vi "Slave FPGA Interface.vi"() -> ()   [LabVIEW 2011]
doc: "This VI shows an example of how to implement a closed loop position move using the NI 9505. The position loop is implemented using PID. The output of the loop is used as the command for the current loop, which then sets the PWM duty cycle for the motor. This example assumes that an encoder is connected for position and velocity feedback. This example does not implement advanced motion features such as trajectory generation and splining."
uses:
  <vilib>/LabVIEW Targets/FPGA/cRIO/cRIO-9505/controls.llb/_nicrio_cRIO-9505_DriveStatus.ctl
  <vilib>/Platform/TimedLoop/XDataNode/timing_clust.ctl
  <vilib>/Platform/TimedLoop/XDataNode/nitl_modes.ctl
  <vilib>/Platform/TimedLoop/XDataNode/wakeup.ctl
  <vilib>/LabVIEW Targets/FPGA/cRIO/shared/nicrio_ModuleControls/nicrio_cRIO-9205_VoltageRange.ctl
  <vilib>/LabVIEW Targets/FPGA/cRIO/shared/nicrio_ModuleControls/nicrio_cRIO-9205_TerminalMode.ctl
  <vilib>/LabVIEW Targets/FPGA/cRIO/cRIO-9505/controls.llb/_nicrio_cRIO-9505_DriveDirection.ctl
  Instance           1 55Saved   Position Control (closed loop) - NI 9505 (FPGA) .vi
  <vilib>/rvi/eio/common/nirviEmuTemplateMethod_errors.vi
  Instance           2 55Saved   Position Control (closed loop) - NI 9505 (FPGA) .vi
  <vilib>/rvi/eio/common/nirviEmuTemplatePropertyGet_noerrors.vi
  Instance           3 55Saved   Position Control (closed loop) - NI 9505 (FPGA) .vi
  <vilib>/Platform/TimedLoop/XDataNode/XDataNode.xnode
  <vilib>/eio/EIONode/EIONode.xnode
  <vilib>/eio/EIOMethodNode/EIOMethodNode.xnode
  <vilib>/eio/EIOPropertyNode/EIOPropertyNode.xnode
  <vilib>/Platform/TimedLoop/XDataNode/XDNodeRunTimeDep.lvlib
  <vilib>/rvi/eio/common/nirviEmuTemplatePropertyGet_errors.vi
  <vilib>/rvi/eio/common/nirviEmuTemplatePropertySet_errors.vi
  <vilib>/rvi/eio/common/nirviEmuTemplatePropertySet_noerrors.vi
panel:
  out "Position Error Status":bool
  out "Position Error Read":i16
  out "Current Command":i16
  in  "Position PID Gains":T1={"Kp"=50, "Kd"=1000, "Ki"=0, "ILim"=1000, "Kv"=0, "Vff"=0, "Aff"=0, "Td"=0}
  in  "Position Loop Rate (usec)":u32
  in  "Position Error Limit":i16
  in  "Position Setpoint":i32
  out "ForceSensor AI0-5":fxp<+/-,26,5>[](array[numeric])
  out "FPGA\nError Out":errorcluster
  in  "Force Loop Rate (usec)":u32=50
  out "Vsup Present":bool
  out "Drive Fault":bool
  out "Drive Status":T2=enum."Disabled"
  out "Temp Fault":bool
  in  "Enable\nDrive":bool
  in  "Disable\nDrive":bool
  in  "Reset Position":bool
  in  "Reset Position Value":i32
  out "Encoder Position":i32
  out "ticks/count":u32
  out "Index (Z) Position":i32
  out "counts (no reset)":i32
  in  "Current PI Gains":T3={"Proportional Gain"=20, "Integral Gain"=10, "Derivative Gain"=0}
  in  "Current Limit":i16 caption="Setpoint"
  in  "Current Loop\nRate (usec)":u32=50
  in  "Trig AI":bool
  in  "Current Feedback":i16
  out "Current Loop Output":i16
  # "VI Execution\nThis VI should be run with \"Position Control (closed loop) - NI 9505 (RT).vi\"."
  # "These parameters control the response of the position loop. Position Setpoint is the desired position to go to. Position Error Limit is the maximum allowed error the setpoint and actual position returned by the encoder loop."
  # "These parameters control the response\nof the current loop. The current limit is the \nmaximum current allowed."
  # "Current Loop Parameters"
  # "Use the Reset Position control to reset the quadrature count to the value in Reset Position Value."
  # "These status controls/indicators are used to enable/disable the drive and read fault information."
  # "Drive Status"
  # "Encoder Parameters"
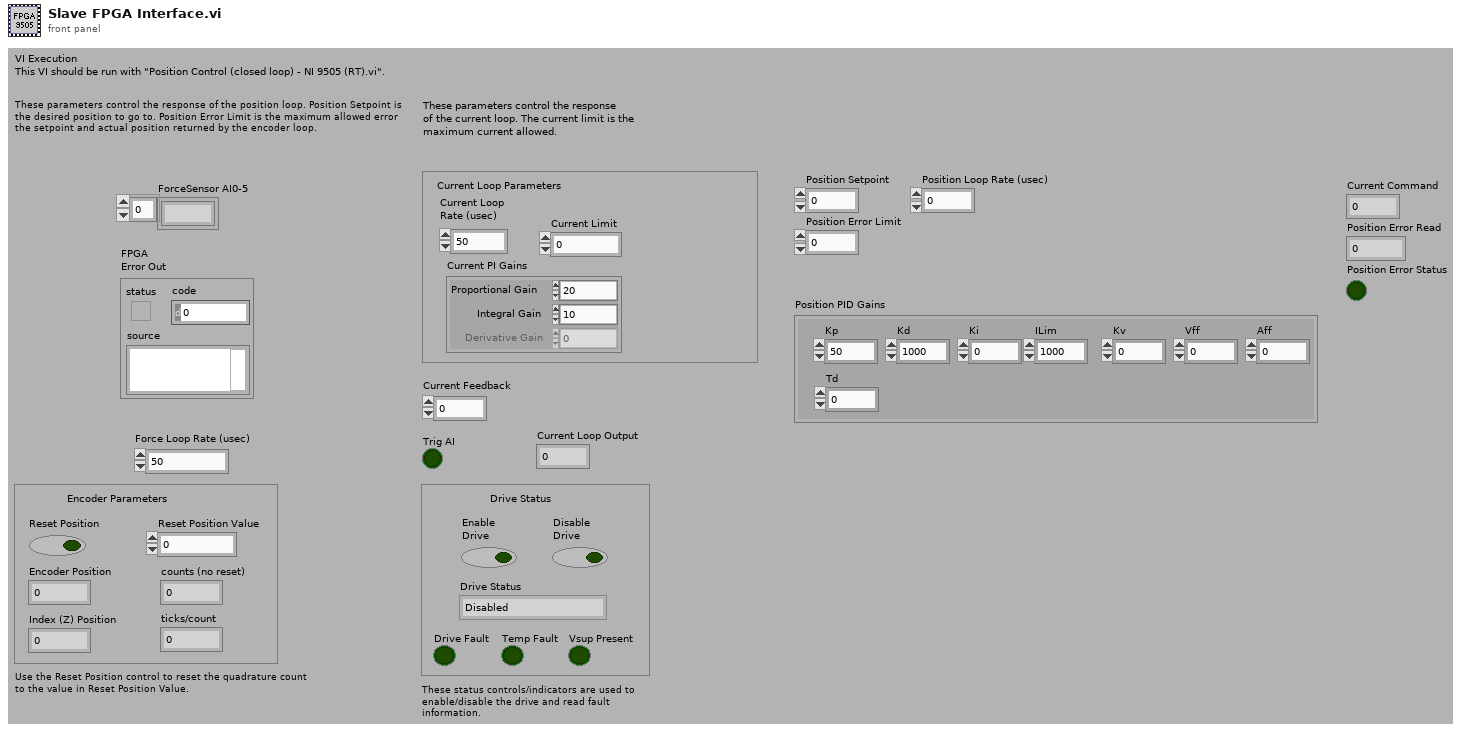
[diagram p1: front panel]
types:
  T1 = cluster{"Kp":i16, "Kd":i16, "Ki":i16, "ILim":i16, "Kv":i16, "Vff":i16, "Aff":i16, "Td":i16}
  T2 = typedef "_nicrio_cRIO-9505_DriveStatus.ctl" = enum8{"Enabled", "Disabled", "Disabled by Drive Fault", "Disabled by Temp. Fault", "Disabled by E-Stop", "Unknown"}
  T3 = cluster{"Proportional Gain":i16, "Integral Gain":i16, "Derivative Gain":i16}
  T4 = typedef "XDNodeRunTimeDep.lvlib/timing_clust.ctl" = cluster{"Expected End [f-1]":u64, "Actual End [f-1]":u64, "Finished Late? [f-1]":bool, "Expected End [i-1]":u64, "Actual End [i-1]":u64, "Finished Late? [i-1]":bool, "Expected Start [i]":u64, "Actual Start [i]":u64, "Expected Start [f]":u64, "Actual Start [f]":u64, "Source Name":string, "Structure Name":string, "Period":i64, "Deadline":i64, "Offset":i64, "Start":i64, "Priority":i32, "Timeout":i32, "Mode":T5, "Wakeup Reason":T6, "Error":errorcluster, "Source Type":string, "Secondary Source Type":string, "Global End Time":u64, "Global Start Time":u64, "Frame Duration":u64, "Iteration Duration":u64, "Assigned CPU":i32, "I/O Scan Engine Mode":u32}
  T5 = typedef "XDNodeRunTimeDep.lvlib/nitl_modes.ctl" = enum32{"No Change", "Process missed periods, maintain original phase", "Discard missed periods, maintain original phase", "Process missed periods, ignore original phase", "Discard missed periods, ignore original phase"}
  T6 = typedef "XDNodeRunTimeDep.lvlib/wakeup.ctl" = enum32{"Normal", "Aborted", "Asynchronous wakeup", "Timing source error", "Timed loop error", "Timeout"}
  T7 = typedef "_nicrio_cRIO-9505_DriveDirection.ctl" = enum8{"Clockwise", "Counterclockwise"}
  T8 = typedef "nicrio_cRIO-9205_VoltageRange.ctl" = enum8{"+/- 10V", "+/- 5V", "+/- 1V", "+/- 200mV"}
  T9 = typedef "nicrio_cRIO-9205_TerminalMode.ctl" = enum8{"RSE", "NRSE", "DIFF"}
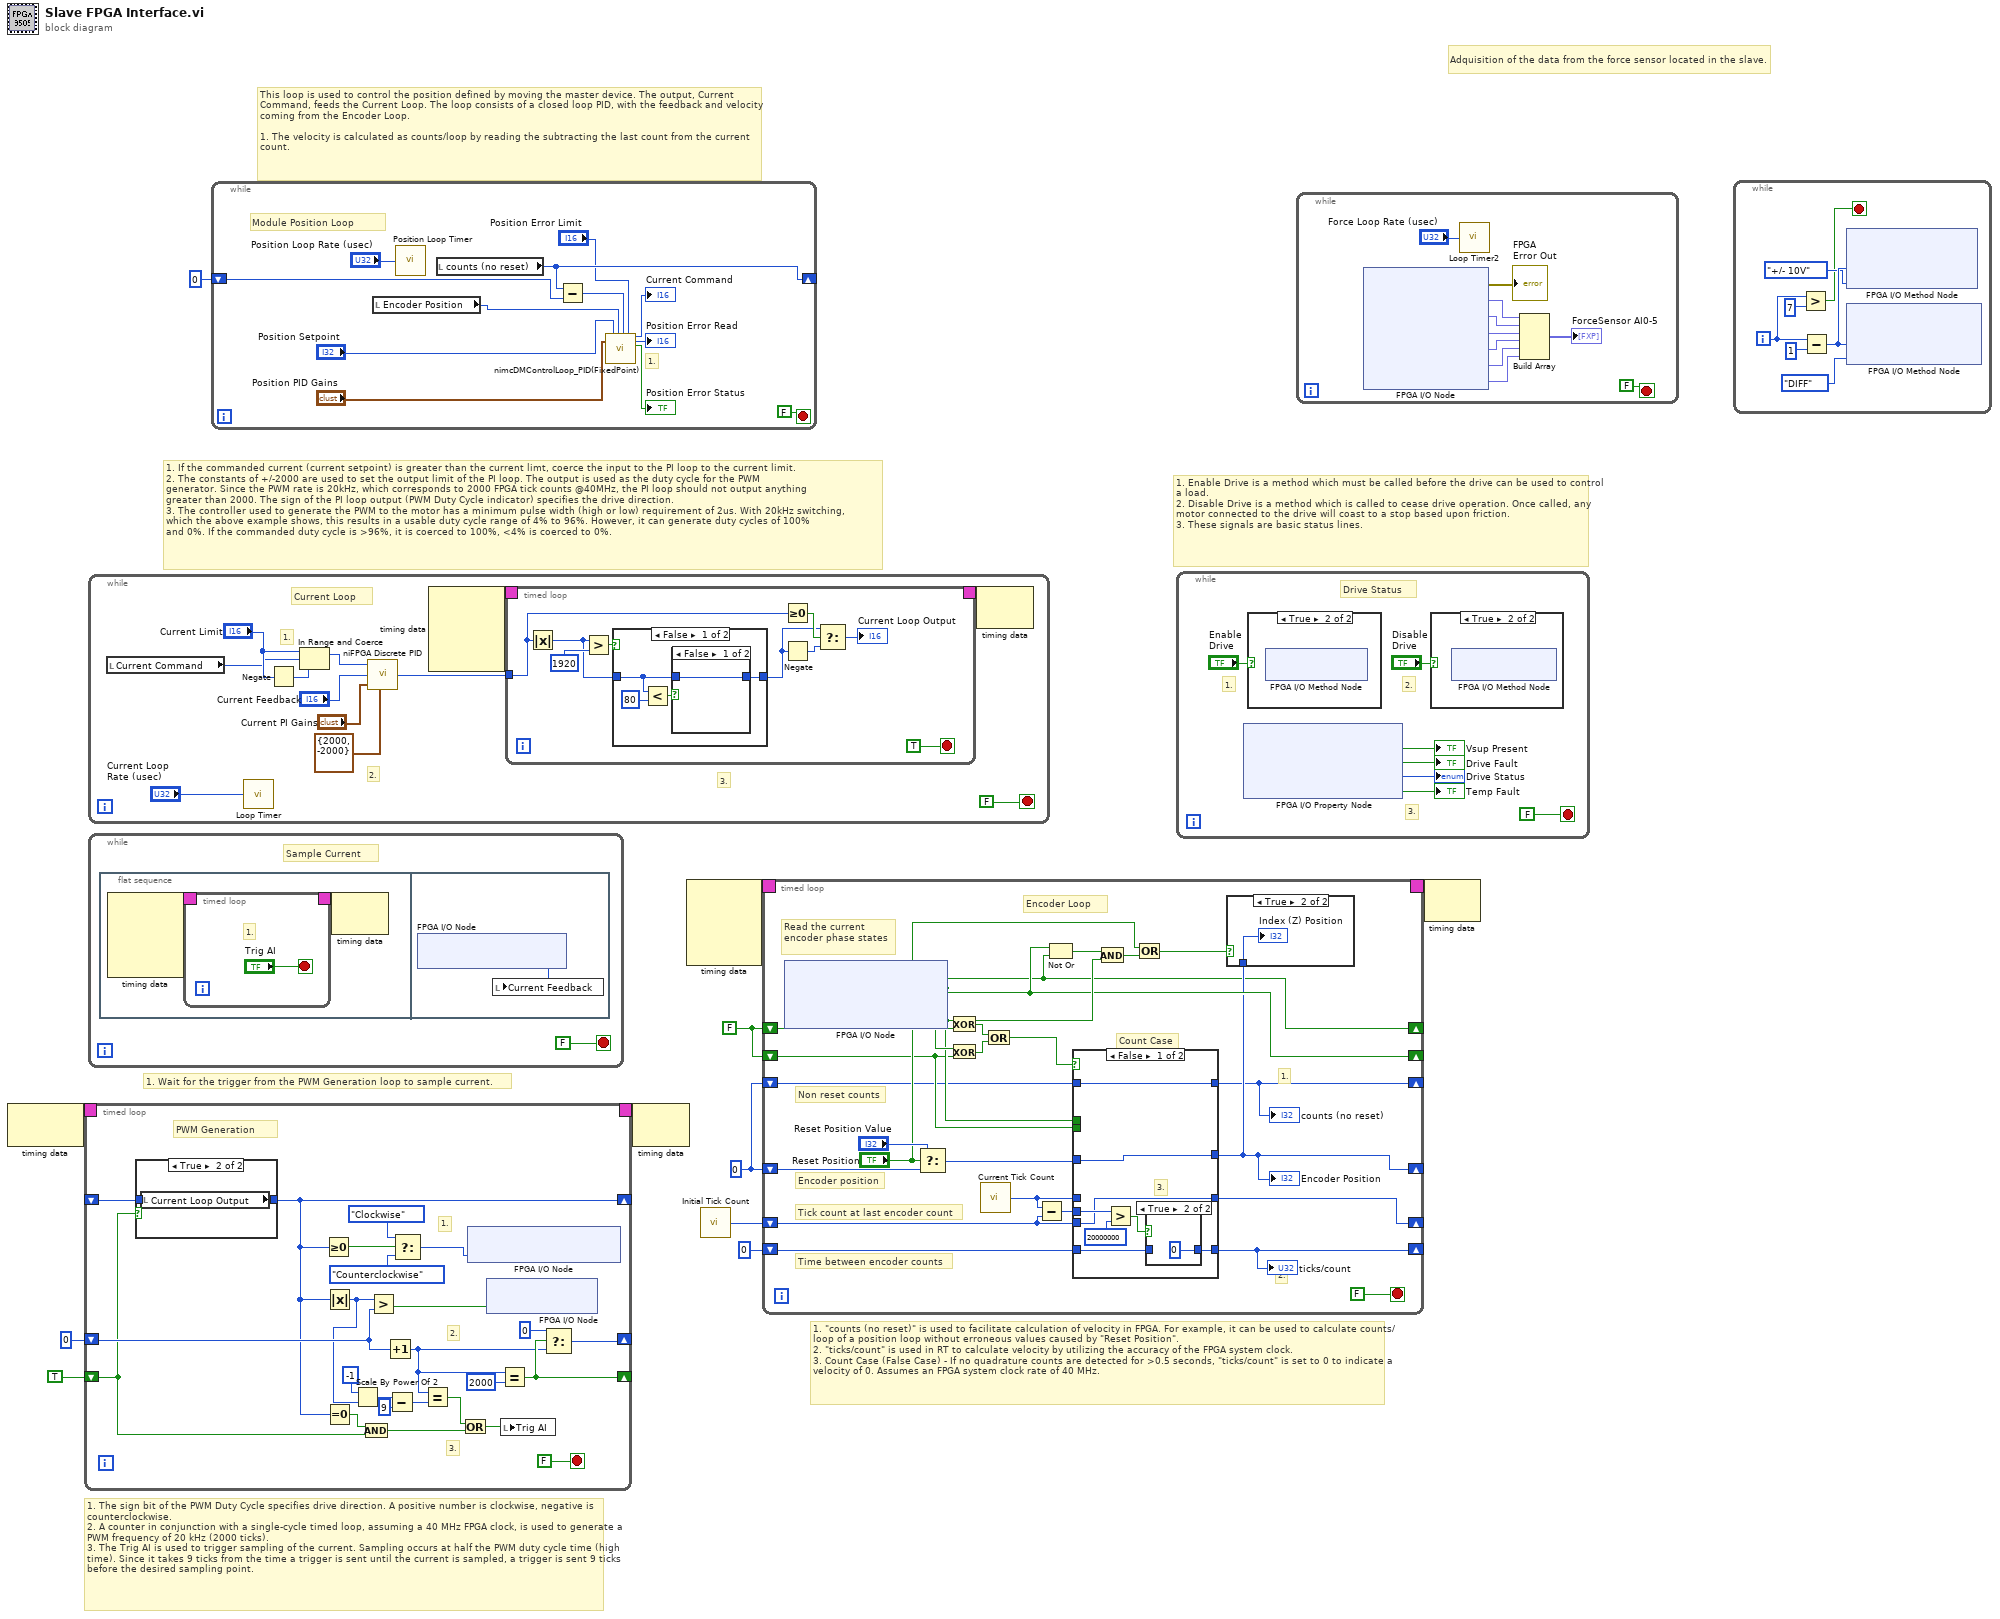
[diagram p0: block diagram]
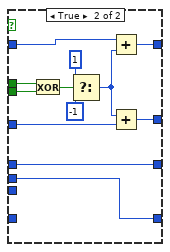
[diagram p4: hidden frame]
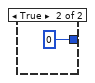
[diagram p6: hidden frame]
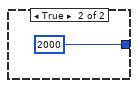
[diagram p7: hidden frame]
diagram:
  w2 = 0 ("Reset Position Value")
  w5 = FALSE ("Encoder Phase A")
  # "This loop is used to control the position defined by moving the master device. The output, Current Command, feeds the Current Loop. The loop consists of a closed loop PID, with the feedback and velocity coming from the Encoder Loop.\n\n1. The velocity is calculated as counts/loop by reading the subtracting the last count from the current count."
  # "Adquisition of the data from the force sensor located in the slave."
  # "1. \"counts (no reset)\" is used to facilitate calculation of velocity in FPGA. For example, it can be used to calculate counts/loop of a position loop without erroneous values caused by \"Reset Position\". \n2. \"ticks/count\" is used in RT to calculate velocity by utilizing the accuracy of the FPGA system clock.\n3. Count Case (False Case) - If no quadrature counts are detected for >0.5 seconds, \"ticks/count\" is set to 0 to indicate a velocity of 0. Assumes an FPGA system clock rate of 40 MHz."
  # "1. Enable Drive is a method which must be called before the drive can be used to control a load.\n2. Disable Drive is a method which is called to cease drive operation. Once called, any motor connected to the drive will coast to a stop based upon friction.\n3. These signals are basic status lines."
  # "1. The sign bit of the PWM Duty Cycle specifies drive direction. A positive number is clockwise, negative is counterclockwise. \n2. A counter in conjunction with a single-cycle timed loop, assuming a 40 MHz FPGA clock, is used to generate a PWM frequency of 20 kHz (2000 ticks).\n3. The Trig AI is used to trigger sampling of the current. Sampling occurs at half the PWM duty cycle time (high time). Since it takes 9 ticks from the time a trigger is sent until the current is sampled, a trigger is sent 9 ticks before the desired sampling point."
  # "1. Wait for the trigger from the PWM Generation loop to sample current."
  # "1. If the commanded current (current setpoint) is greater than the current limt, coerce the input to the PI loop to the current limit.\n2. The constants of +/-2000 are used to set the output limit of the PI loop. The output is used as the duty cycle for the PWM\ngenerator. Since the PWM rate is 20kHz, which corresponds to 2000 FPGA tick counts @40MHz, the PI loop should not output anything\ngreater than 2000. The sign of the PI loop output (PWM Duty Cycle indicator) specifies the drive direction.\n3. The controller used to generate the PWM to the motor has a minimum pulse width (high or low) requirement of 2us. With 20kHz switching,\nwhich the above example shows, this results in a usable duty cycle range of 4% to 96%. However, it can generate duty cycles of 100%\nand 0%. If the commanded duty cycle is >96%, it is coerced to 100%, <4% is coerced to 0%."
  n1 = node-c288() -> (w11:T4)  [unwired: 1 out]
  n2 = timed-loop {
    timing: w11 -> [_]
    timing-out: [_] -> w10
    shift-right: [w32] -> _
    shift-left: i16 0 -> [w35]
    shift-right: [w31] -> _
    shift-left: TRUE -> [w28]
    shift-right: [w16] -> _
    shift-left: _ -> [w30]
    stop <- FALSE stop-if-true
    # "3."
    # "2."
    # "1."
    # "PWM Generation"
    n3 = case shown="True" w28 {
      tunnel: [w36 w37] -> w16
      tunnel: w30 -> [w36 _]
      frame False {
      }
      frame True {
        n4 = local read "Current Loop Output"() -> (w37:i16)
      }
    }
    n5 = Greater Or Equal To 0?(x=w16) -> (x >= 0?=w24:bool)
    n6 = Absolute Value(x=w16) -> (abs(x)=w14:i16)
    n7 = Equal To 0?(x=w16) -> (x = 0?=w29:bool)
    n8 = Scale By Power Of 2(n=i8 -1, x=w14) -> (x*2^n=w18:i16)
    n9 = And(x=w29, y=w28) -> (x .and. y?=w25:bool)
    n10 = Greater?(x=w14, y=w35) -> (0:w13:bool)
    n11 = Increment(x=w35) -> (x+1=w27:i16)
    n12 = Subtract(x=w18, y=i8 9) -> (x-y=w17:i16)
    n13 = Select(t=_nicrio_cRIO-9505_DriveDirection."Clockwise" ("Drive Direction"), s=w24, f=_nicrio_cRIO-9505_DriveDirection."Counterclockwise" ("Drive Direction")) -> (s? t:f=w12:T7)
    n14 = Equal?(x=w27, y=w17) -> (x = y?=w26:bool)
    n15 = Or(x=w26, y=w25) -> (x .or. y?=w20:bool)
    n16 = xnode "FPGA I/O Node"("Motor/Drive Direction"=w12) -> ()  [unwired: 1 in, 1 out]
    n17 = xnode "FPGA I/O Node"("Motor/Motor"=w13) -> ()  [unwired: 1 in, 1 out]
    n18 = Equal?(x=w27, y=i16 2000) -> (x = y?=w31:bool)
    n19 = local write "Trig AI"(w20) -> ()
    n20 = Select(t=i16 0, s=w31, f=w27) -> (s? t:f=w32:i16)
  }
  n21 = while {
    stop <- FALSE stop-if-true
    # "3."
    # "2."
    # "1."
    # "Current Loop"
    n22 = local read "Current Command"() -> (w40:i16)
    n23 = call "Loop Timer"("Count(uSec)"="Current Loop\nRate (usec)") -> ()  [unwired: 1 out]
    n24 = Negate(x="Current Limit") -> (-x=w44:i16)
    n25 = In Range and Coerce(upper limit="Current Limit", x=w40, lower limit=w44) -> (coerced(x)=w42:i16)  [unwired: 1 out]
    n26 = call <vilib>:"niFPGA Discrete PID.vi"("setpoint"=w42, "process variable"="Current Feedback", "PID gains (x 2^8)"="Current PI Gains", "output range"=cluster{"output high":i16, "output low":i16} {"output high"=2000, "output low"=-2000}) -> ("output"=w47:i16)  [unwired: 1 in, 4 out]
    n27 = node-c288() -> (w46:T4)  [unwired: 4 out]
    n28 = timed-loop {
      timing: w46 -> [_]
      timing-out: [_] -> w45
      tunnel: w47 -> [w54]
      stop <- TRUE stop-if-true
      n29 = Absolute Value(x=w54) -> (abs(x)=w55:i16)
      n30 = Greater?(x=w55, y=i16 1920 ("upper limit")) -> (0:w57:bool)
      n31 = case shown="False" w57 {
        tunnel: [w63 i16 2000 ("upper limit")] -> w56
        tunnel: w55 -> [w61 _]
        frame False {
          n32 = Less?(x=w61, y=i16 80 ("lower limit")) -> (x < y?=w62:bool)
          n33 = case shown="False" w62 {
            tunnel: [w65 i16 0 ("upper limit")] -> w63
            tunnel: w61 -> [w65 _]
            frame False {
            }
            frame True {
            }
          }
        }
        frame True {
        }
      }
      n34 = Greater Or Equal To 0?(x=w54) -> (x >= 0?=w60:bool)
      n35 = Negate(x=w56) -> (-x=w59:i16)
      n36 = Select(t=w56, s=w60, f=w59) -> (s? t:f=→"Current Loop Output":i16)
    }
    n37 = node-c288(w45) -> ()  [unwired: 1 out]
  }
  n38 = while {
    stop <- FALSE stop-if-true
    # "Sample Current"
    n39 = flat-sequence {
      frame #0 {
        n40 = node-c288() -> (w74:T4)  [unwired: 4 out]
        n41 = timed-loop {
          timing: w74 -> [_]
          timing-out: [_] -> w73
          stop <- "Trig AI" stop-if-true
          # "1."
        }
        n42 = node-c288(w73) -> ()  [unwired: 1 out]
      }
      frame #1 {
        n43 = xnode "FPGA I/O Node"() -> ("Motor/Current Sense"=w80:i16)  [unwired: 1 in, 1 out]
        n44 = local write "Current Feedback"(w80) -> ()
      }
    }
  }
  n45 = while "Position Control Loop" {
    shift-right: [w89] -> _
    shift-left: 0 ("Encoder Position") -> [w88]
    stop <- FALSE stop-if-true
    # "1."
    # "Module Position Loop"
    n46 = local read "Encoder Position"() -> (w81:i32)
    n47 = call "Position Loop Timer"("Count(uSec)"="Position Loop Rate (usec)") -> ()  [unwired: 1 out]
    n48 = local read "counts (no reset)"() -> (w89:i32)
    n49 = Subtract(x=w89, y=w88) -> (x-y=w90:i32)
    n50 = call "nimcDMControlLoop_PID(FixedPoint).vi"("PID Gains"="Position PID Gains", "Setpoint"="Position Setpoint", "Position Feedback"=w81, "Velocity Feedback"=w90, "Position Error Limit"="Position Error Limit") -> ("Output"=→"Current Command":i16, "Position Error Read"=→"Position Error Read":i16, "Position Error Status"=→"Position Error Status":bool)  [unwired: 2 in, 10 out]
  }
  n51 = node-c288(w10) -> ()  [unwired: 1 out]
  n52 = node-c288() -> (w7:T4)  [unwired: 4 out]
  n53 = call "Initial Tick Count"() -> ("Tick Count(Ticks)"=w4:u32)
  n54 = timed-loop {
    shift-right: [w99] -> _
    shift-left: w5 -> [w117]
    shift-right: [w105] -> _
    shift-left: w5 -> [w98]
    shift-right: [w101] -> _
    shift-left: w2 -> [w114]
    shift-right: [w110] -> _
    shift-left: w4 -> [w94]
    shift-right: [w109] -> _
    shift-left: u32 0 -> [w108]
    timing: w7 -> [_]
    timing-out: [_] -> w6
    shift-right: [w96] -> _
    shift-left: w2 -> [w97]
    stop <- FALSE stop-if-true
    # "Count Case"
    # "Encoder Loop"
    # "2."
    # "1."
    # "Read the current\nencoder phase states"
    # "Non reset counts"
    # "Encoder position"
    # "Time between encoder counts"
    # "Tick count at last encoder count"
    n55 = xnode "FPGA I/O Node"() -> ("Motor/Encoder Phase A"=w99:bool, "Motor/Encoder Phase B"=w105:bool, "Motor/Encoder Index"=w106:bool)  [unwired: 3 in, 3 out]
    n56 = Select(t="Reset Position Value", s="Reset Position", f=w114) -> (s? t:f=w112:i32)
    n57 = Exclusive Or(1:w117, 2:w99) -> (0:w116:bool)
    n58 = Exclusive Or(1:w98, 2:w105) -> (0:w115:bool)
    n59 = call "Current Tick Count"() -> ("Tick Count(Ticks)"=w95:u32)
    n60 = Or(x=w116, y=w115) -> (x .or. y?=w113:bool)
    n61 = Subtract(x=w95, y=w94) -> (x-y=w93:u32)
    n62 = Not Or(1:w99, 2:w105) -> (0:w103:bool)
    n63 = case shown="False" w113 {
      tunnel: [w126 w134] -> w101
      tunnel: w112 -> [w126 w140]
      tunnel: w95 -> [_ w130]
      tunnel: [w121 w130] -> w110
      tunnel: w94 -> [w121 _]
      tunnel: [w119 w129] -> w109
      tunnel: w108 -> [w120 _]
      tunnel: w99 -> [_ w136]
      tunnel: w98 -> [_ w135]
      tunnel: [w125 w132] -> w96
      tunnel: w97 -> [w125 w131]
      tunnel: w93 -> [w122 w129]
      frame False {
        # "3."
        n64 = Greater?(x=w122, y=20000000 ("x")) -> (0:w123:bool)
        n65 = case shown="True" w123 {
          tunnel: [w127 u32 0] -> w119
          tunnel: w120 -> [w127 _]
          frame False {
          }
          frame True {
          }
        }
      }
      frame True {
        n66 = Exclusive Or(1:w135, 2:w136) -> (0:w137:bool)
        n67 = Select(t=1 ("16 bit"), s=w137, f=-1 ("16 bit")) -> (s? t:f=w133:i32)
        n68 = Add(x=w131, y=w133) -> (x+y=w132:i32)
        n69 = Add(x=w133, y=w140) -> (x+y=w134:i32)
      }
    }
    "Encoder Position" <- w101
    "ticks/count" <- w109
    "counts (no reset)" <- w96
    n70 = And(x=w103, y=w106) -> (x .and. y?=w104:bool)
    n71 = Or(x="Reset Position", y=w104) -> (x .or. y?=w102:bool)
    n72 = case shown="True" w102 {
      tunnel: w101 -> [_ w118]
      frame False {
      }
      frame True {
        "Index (Z) Position" <- w118
      }
    }
  }
  n73 = while {
    stop <- FALSE stop-if-true
    # "Drive Status"
    # "3."
    # "2."
    # "1."
    n74 = xnode "FPGA I/O Property Node"() -> ("Vsup Present"=→"Vsup Present":bool, "Drive Fault"=→"Drive Fault":bool, "Drive Status"=→"Drive Status":T2, "Over Temperature Fault"=→"Temp Fault":bool)  [unwired: 1 in, 1 out]
    n75 = case shown="True" "Enable\nDrive" {
      frame False {
      }
      frame True {
        n76 = xnode "FPGA I/O Method Node"() -> ()  [unwired: 1 in, 1 out]
      }
    }
    n77 = case shown="True" "Disable\nDrive" {
      frame False {
      }
      frame True {
        n78 = xnode "FPGA I/O Method Node"() -> ()  [unwired: 1 in, 1 out]
      }
    }
  }
  n79 = while {
    stop <- FALSE stop-if-true
    n80 = xnode "FPGA I/O Node"() -> ("error out"=→"FPGA\nError Out":errorcluster, "ForceSensor/AI0"=w155:fxp<+/-,26,5>, "ForceSensor/AI1"=w156:fxp<+/-,26,5>, "ForceSensor/AI2"=w157:fxp<+/-,26,5>, "ForceSensor/AI3"=w158:fxp<+/-,26,5>, "ForceSensor/AI4"=w154:fxp<+/-,26,5>, "ForceSensor/AI5"=w153:fxp<+/-,26,5>)  [unwired: 7 in, 6 out]
    n81 = call "Loop Timer2"("Count(uSec)"="Force Loop Rate (usec)") -> ()  [unwired: 1 out]
    n82 = Build Array(w155, w156, w157, w158, w154, w153) -> (→"ForceSensor AI0-5":fxp<+/-,26,5>[])
  }
  n83 = node-c288(w6) -> ()  [unwired: 1 out]
  n84 = while {
    i -> [w163]
    stop <- w160 stop-if-true
    n85 = Greater?(x=w163, y=7) -> (0:w160:bool)
    n86 = Subtract(x=w163, y=1) -> (x-y=w162:i32)
    n87 = xnode "FPGA I/O Method Node"("AI Channel"=w162, "Voltage Range"=nicrio_cRIO-9205_VoltageRange."+/- 10V") -> ()  [unwired: 1 in, 1 out]
    n88 = xnode "FPGA I/O Method Node"("AI Channel"=w162, "Terminal Mode"=nicrio_cRIO-9205_TerminalMode."DIFF") -> ()  [unwired: 1 in, 1 out]
  }
